vi "filter.vi"(8 "debug":bool, 9 "conf.valid":bool, 10 "conf":u64, 11 "reset":bool) -> (1 "Ready.for.OrderBook.Command.Input":bool, 2 "Ready.for.Configuration.Input":bool)   [LabVIEW 2020]
uses:
  filter.states.ctl
  filter.data.ctl
  filter.data.scratch.ctl
  order.slot.ctl
  ticker.slot.ctl
  filter.memory.command.ctl
  filter.debug.ctl
  filter.debug.slot.ctl
  Market.Data.Common/fpga/orderbook.command.ctl
  Market.Data.Common/fpga/fpganow.common.fpga.lvlib
  filter.state.slot.ctl
  filter.state.ctl
  Market.Data.Common/fpga/orderbook.command.type.ctl
  order.slot.hm.ctl
  order.slot.access.ctl
  ticker.slot.access.ctl
  filter.hash.ctl
  Filter.lvclass
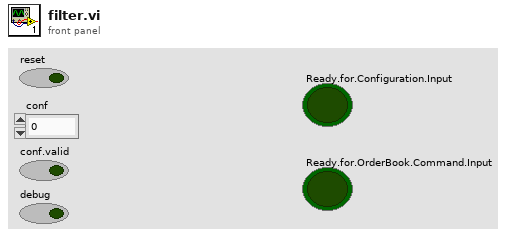
[diagram p1: front panel]
types:
  T1 = typedef "filter.data.ctl" = cluster{"filter.state":T2, "number.of.tickers":u32, "filter.saved.state":T2, "Send.Command":bool, "hash.1":T3, "hash.2":T3, "Scratch":T4, "debug":T5, "mem.cmd":T7, "get.state":T13, "ob.cmd":T15, "number.of.orders":u32, "Filter.lvclass":refnum<class "Filter.lvclass">, "counter":i16}
  T2 = typedef "filter.states.ctl" = enum16{"Noop", "Reset", "Debug", "Configuration", "Wait.for.Command", "Filter.Add", "Filter.Other", "Insert.Order", "Delete Order", "Get.State", "Get.Watchlist", "Get.Memory"}
  T3 = typedef "filter.hash.ctl" = cluster{"req":bool, "data.in":u64, "crc32.out":u32}
  T4 = typedef "filter.data.scratch.ctl" = cluster{"I":u32, "N":u32, "Mode":u32, "OrderId":u64, "First Call?":bool, "Just Write":bool, "left":u32, "right":u32, "Reset":bool}
  T5 = typedef "filter.debug.ctl" = cluster{"write":bool, "v":T6}
  T6 = typedef "filter.debug.slot.ctl" = cluster{"slot.0":u64, "slot.1":u64, "slot.2":u64, "slot.3":u64}
  T7 = typedef "filter.memory.command.ctl" = cluster{"Read Order Request":bool, "Write Order Request":bool, "Read Order Valid":bool, "Write Order Address":u32, "Read Order Address":u32, "order.slot.value":T8, "ticker":T9, "ord.1":T11, "ord.2":T11}
  T8 = typedef "order.slot.ctl" = cluster{"OrderId":u64, "Quantity":u64}
  T9 = typedef "ticker.slot.access.ctl" = cluster{"read.req":bool, "write.req":bool, "read.valid":bool, "read.addr":u32, "write.addr":u32, "v":T10}
  T10 = typedef "ticker.slot.ctl" = cluster{"Symbol":u64}
  T11 = typedef "order.slot.access.ctl" = cluster{"read.req":bool, "write.req":bool, "read.valid":bool, "read.addr":u32, "write.addr":u32, "v":T12}
  T12 = typedef "order.slot.hm.ctl" = cluster{"OrderId":u64, "Quantity":u64, "IsValid":bool}
  T13 = typedef "filter.state.ctl" = cluster{"write.req":bool, "v":T14}
  T14 = typedef "filter.state.slot.ctl" = cluster{"OrderId":u64, "Quantity":u64}
  T15 = typedef "fpganow.common.fpga.lvlib/orderbook.command.ctl" = cluster{"type":T16, "side":u8, "orderId ":u64, "quantity":u32, "symbol":u64, "price":u64, "executed.qty":u32, "canceled.qty":u32, "remaining.qty":u32, "seconds":u64, "nanoseconds":u64, "Add":bool, "Edit":bool, "Remove":bool, "seq no":u32, "recv.time":u64, "parse.time":u64}
  T16 = typedef "fpganow.common.fpga.lvlib/orderbook.command.type.ctl" = enum8{"Time", "AddOrder", "OrderExecuted", "OrderExecutedAtPrice", "ReduceSize", "ModifyOrder", "DeleteOrder", "Get.Everything", "Get.All.Orders", "Get.Top"}
  T17 = cluster{"reset":bool, "conf":u64, "conf.valid":bool, "debug":bool}
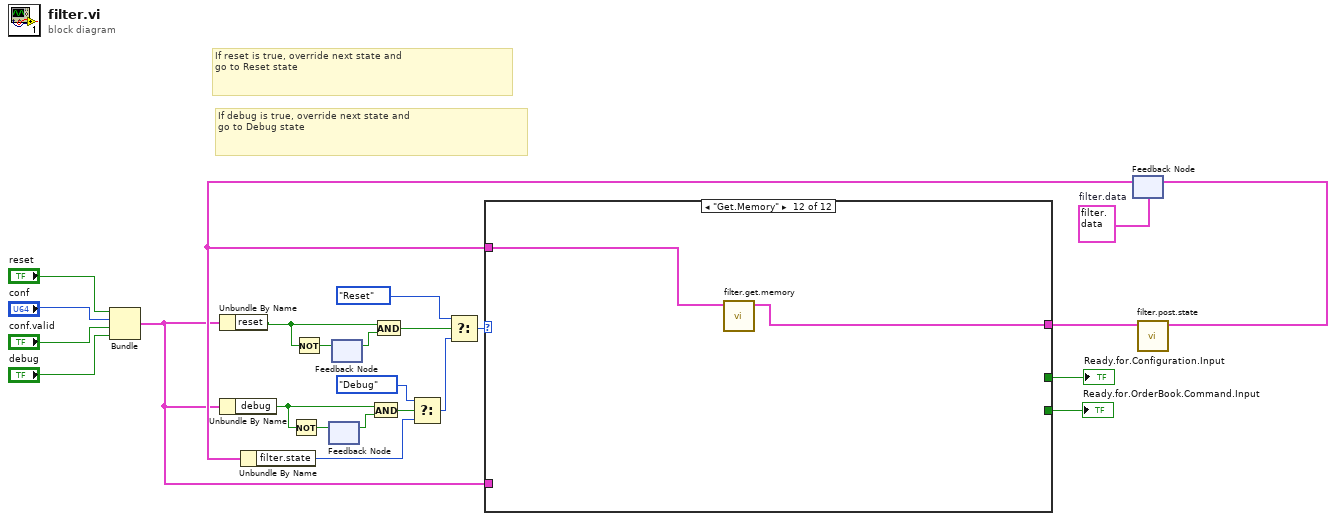
[diagram p0: block diagram]
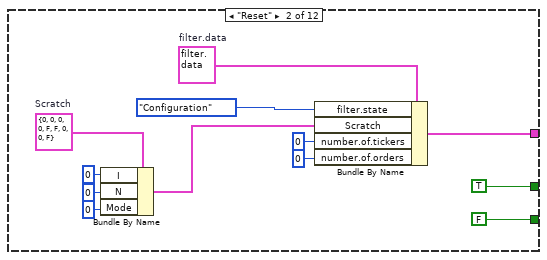
[diagram p3: hidden frame]
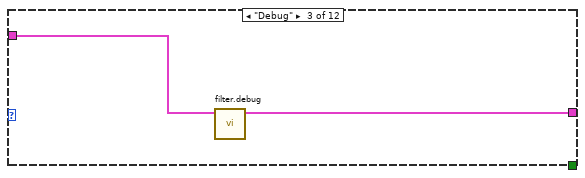
[diagram p4: hidden frame]
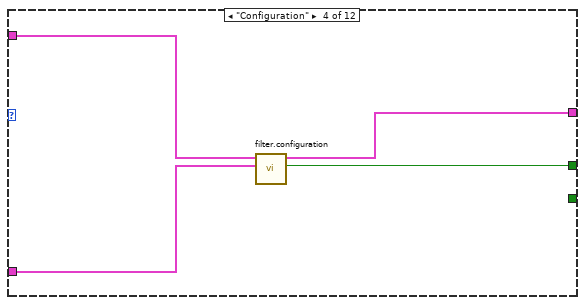
[diagram p5: hidden frame]
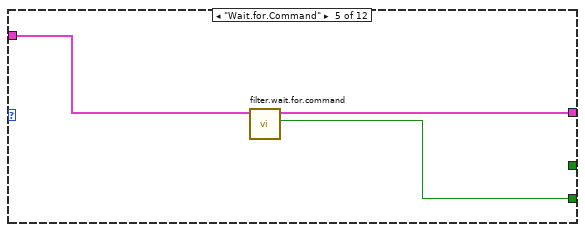
[diagram p6: hidden frame]
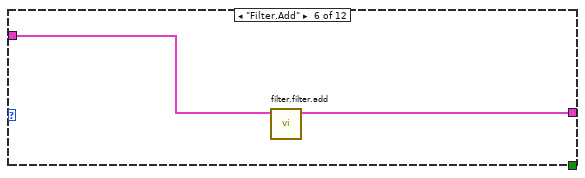
[diagram p7: hidden frame]
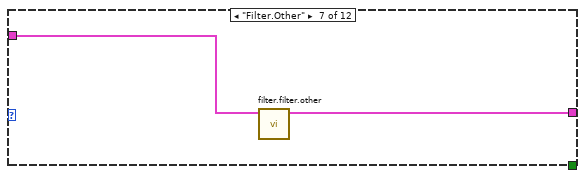
[diagram p8: hidden frame]
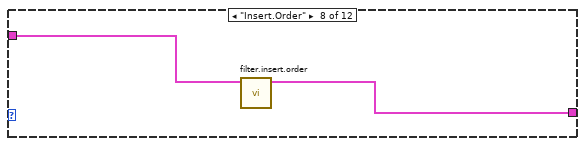
[diagram p9: hidden frame]
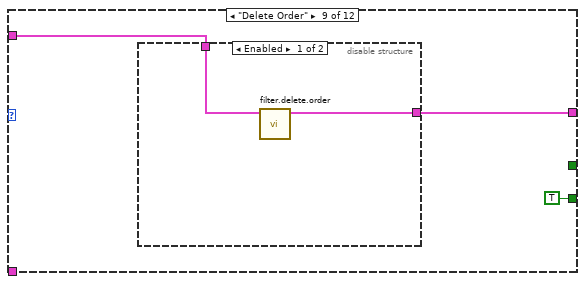
[diagram p10: hidden frame]
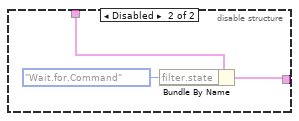
[diagram p11: hidden frame]
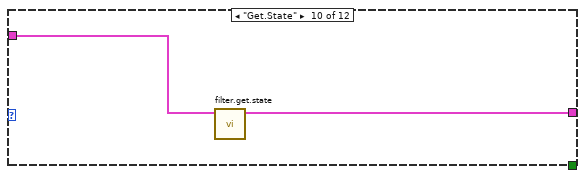
[diagram p12: hidden frame]
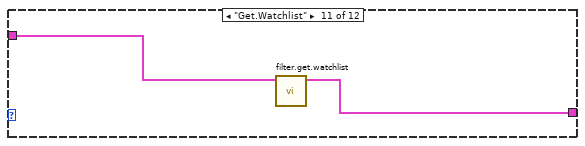
[diagram p13: hidden frame]
diagram:
  w9 = T1 {"filter.state"=enum."Noop", "number.of.tickers"=0, "filter.saved.state"=enum."Noop", "Send.Command"=FALSE, "hash.1"={"req"=FALSE, "data.in"=0, "crc32.out"=0}, "hash.2"={"req"=FALSE, "data.in"=0, "crc32.out"=0}, "Scratch"={"I"=0, "N"=0, "Mode"=0, "OrderId"=0, "First Call?"=FALSE, "Just Write"=FALSE, "left"=0, "right"=0, "Reset"=FALSE}, "debug"={"write"=FALSE, "v"={"slot.0"=0, "slot.1"=0, "slot.2"=0, "slot.3"=0}}, "mem.cmd"={"Read Order Request"=FALSE, "Write Order Request"=FALSE, "Read Order Valid"=FALSE, "Write Order Address"=0, "Read Order Address"=0, "order.slot.value"={"OrderId"=0, "Quantity"=0}, "ticker"={"read.req"=FALSE, "write.req"=FALSE, "read.valid"=FALSE, "read.addr"=0, "write.addr"=0, "v"={"Symbol"=0}}, "ord.1"={"read.req"=FALSE, "write.req"=FALSE, "read.valid"=FALSE, "read.addr"=0, "write.addr"=0, "v"={"OrderId"=0, "Quantity"=0, "IsValid"=FALSE}}, "ord.2"={"read.req"=FALSE, "write.req"=FALSE, "read.valid"=FALSE, "read.addr"=0, "write.addr"=0, "v"={"OrderId"=0, "Quantity"=0, "IsValid"=FALSE}}}, "get.state"={"write.req"=FALSE, "v"={"OrderId"=0, "Quantity"=0}}, "ob.cmd"={"type"=enum."Time", "side"=0, "orderId "=0, "quantity"=0, "symbol"=0, "price"=0, "executed.qty"=0, "canceled.qty"=0, "remaining.qty"=0, "seconds"=0, "nanoseconds"=0, "Add"=FALSE, "Edit"=FALSE, "Remove"=FALSE, "seq no"=0, "recv.time"=0, "parse.time"=0}, "number.of.orders"=0, "Filter.lvclass"=refnum, "counter"=0}  # filter.data
  # "If debug is true, override next state and \ngo to Debug state"
  # "If reset is true, override next state and \ngo to Reset state"
  n1 = Bundle("reset"="reset", "conf"="conf", "conf.valid"="conf.valid", "debug"="debug") -> (w3:T17)  [unwired: 1 in]
  n2 = Unbundle By Name(w3) -> ("reset"=w18:bool)
  n3 = Unbundle By Name(w3) -> ("debug"=w15:bool)
  n4 = Not(x=w15) -> (.not. x?=w17:bool)
  n5 = Not(x=w18) -> (.not. x?=w20:bool)
  n6 = feedback #1() -> (w16:bool)  [unwired: 1 in]
  n7 = feedback-in #1(w17) -> ()
  n8 = feedback #2() -> (w19:bool)  [unwired: 1 in]
  n9 = feedback-in #2(w20) -> ()
  n10 = And(x=w15, y=w16) -> (x .and. y?=w12:bool)
  n11 = And(x=w18, y=w19) -> (x .and. y?=w13:bool)
  n12 = feedback #3(w9) -> (w6:T1)
  n13 = Unbundle By Name(w6) -> ("filter.state"=w8:T2)
  n14 = Select(t=filter.states."Debug" ("filter.states"), s=w12, f=w8) -> (s? t:f=w10:T2)
  n15 = Select(t=filter.states."Reset" ("filter.states"), s=w13, f=w10) -> (s? t:f=w7:T2)
  n16 = case shown="\"Get.Memory\"" w7 {
    tunnel: [w25 w36 w39 w43 w44 w48 w49 w51 w53 w62 w63 w65] -> w1
    tunnel: w6 -> [w25 _ w38 w41 w46 w47 w50 w52 w54 w61 w64 w66]
    tunnel: [_ TRUE _ w40 _ _ _ _ _ _ _ _] -> w5
    tunnel: [_ FALSE _ _ w45 _ _ _ TRUE ("Ready.for.OrderBook.Command.Input") _ _ _] -> w4
    tunnel: w3 -> [_ _ _ w42 _ _ _ _ _ _ _ _]
    frame "Noop", Default {
    }
    frame "Reset" {
      w32 = T4 {"I"=0, "N"=0, "Mode"=0, "OrderId"=0, "First Call?"=FALSE, "Just Write"=FALSE, "left"=0, "right"=0, "Reset"=FALSE}  # Scratch
      w37 = T1 {"filter.state"=enum."Noop", "number.of.tickers"=0, "filter.saved.state"=enum."Noop", "Send.Command"=FALSE, "hash.1"={"req"=FALSE, "data.in"=0, "crc32.out"=0}, "hash.2"={"req"=FALSE, "data.in"=0, "crc32.out"=0}, "Scratch"={"I"=0, "N"=0, "Mode"=0, "OrderId"=0, "First Call?"=FALSE, "Just Write"=FALSE, "left"=0, "right"=0, "Reset"=FALSE}, "debug"={"write"=FALSE, "v"={"slot.0"=0, "slot.1"=0, "slot.2"=0, "slot.3"=0}}, "mem.cmd"={"Read Order Request"=FALSE, "Write Order Request"=FALSE, "Read Order Valid"=FALSE, "Write Order Address"=0, "Read Order Address"=0, "order.slot.value"={"OrderId"=0, "Quantity"=0}, "ticker"={"read.req"=FALSE, "write.req"=FALSE, "read.valid"=FALSE, "read.addr"=0, "write.addr"=0, "v"={"Symbol"=0}}, "ord.1"={"read.req"=FALSE, "write.req"=FALSE, "read.valid"=FALSE, "read.addr"=0, "write.addr"=0, "v"={"OrderId"=0, "Quantity"=0, "IsValid"=FALSE}}, "ord.2"={"read.req"=FALSE, "write.req"=FALSE, "read.valid"=FALSE, "read.addr"=0, "write.addr"=0, "v"={"OrderId"=0, "Quantity"=0, "IsValid"=FALSE}}}, "get.state"={"write.req"=FALSE, "v"={"OrderId"=0, "Quantity"=0}}, "ob.cmd"={"type"=enum."Time", "side"=0, "orderId "=0, "quantity"=0, "symbol"=0, "price"=0, "executed.qty"=0, "canceled.qty"=0, "remaining.qty"=0, "seconds"=0, "nanoseconds"=0, "Add"=FALSE, "Edit"=FALSE, "Remove"=FALSE, "seq no"=0, "recv.time"=0, "parse.time"=0}, "number.of.orders"=0, "Filter.lvclass"=refnum, "counter"=0}  # filter.data
      n17 = Bundle By Name(cluster=w32, "I"=u32 0, "N"=u32 0, "Mode"=u32 0) -> (w31:T4)
      n18 = Bundle By Name(cluster=w37, "filter.state"=filter.states."Configuration", "Scratch"=w31, "number.of.tickers"=u32 0, "number.of.orders"=u32 0) -> (w36:T1)
    }
    frame "Debug" {
      n19 = call "filter.debug.vi"("filter.data in"=w38) -> ("filter.data out"=w39:T1)  [unwired: 10 in]
    }
    frame "Configuration" {
      n20 = call "filter.configuration.vi"("Cluster"=w42, "filter.data in"=w41) -> ("Boolean"=w40:bool, "filter.data out"=w43:T1)  [unwired: 8 in]
    }
    frame "Wait.for.Command" {
      n21 = call "filter.wait.for.command.vi"("filter.data in"=w46) -> ("Ready.for.OrderBook.Command.Input"=w45:bool, "filter.data out"=w44:T1)  [unwired: 9 in]
    }
    frame "Filter.Add" {
      n22 = call "filter.filter.add.vi"("filter.data in"=w47) -> ("filter.data out"=w48:T1)  [unwired: 10 in]
    }
    frame "Filter.Other" {
      n23 = call "filter.filter.other.vi"("filter.data in"=w50) -> ("filter.data out"=w49:T1)  [unwired: 10 in]
    }
    frame "Insert.Order" {
      n24 = call "filter.insert.order.vi"("filter.data.in"=w52) -> ("filter.data.out"=w51:T1)  [unwired: 10 in]
    }
    frame "Delete Order" {
      n25 = disable-structure shown="Enabled" {
        disable-tunnel: w54 -> [w57 w60]
        disable-tunnel: [w56 w59] -> w53
        frame Enabled {
          n26 = call "filter.delete.order.vi"("filter.data in"=w57) -> ("filter.data out"=w56:T1)  [unwired: 10 in]
        }
        frame Disabled {
          n27 = Bundle By Name(cluster=w60, "filter.state"=filter.states."Wait.for.Command") -> (w59:T1)
        }
      }
    }
    frame "Get.State" {
      n28 = call "filter.get.state.vi"("filter.data in"=w61) -> ("filter.data out"=w62:T1)  [unwired: 10 in]
    }
    frame "Get.Watchlist" {
      n29 = call "filter.get.watchlist.vi"("filter.data in"=w64) -> ("filter.data out"=w63:T1)  [unwired: 10 in]
    }
    frame "Get.Memory" {
      n30 = call "filter.get.memory.vi"("filter.data in"=w66) -> ("filter.data out"=w65:T1)  [unwired: 10 in]
    }
  }
  "Ready.for.OrderBook.Command.Input" <- w4
  "Ready.for.Configuration.Input" <- w5
  n31 = call "filter.post.state.vi"("filter.data in"=w1) -> ("filter.data out 2"=w2:T1)  [unwired: 10 in]
  n32 = feedback-in #3(w2) -> ()
